vi "OpenStringFormatter Example.vi"() -> ()   [LabVIEW 2020]
uses:
  _built_ppls/OpenStringFormatter.lvlibp/StringFormatter.lvclass
panel:
  out "Value 2":string
  out "Value":string
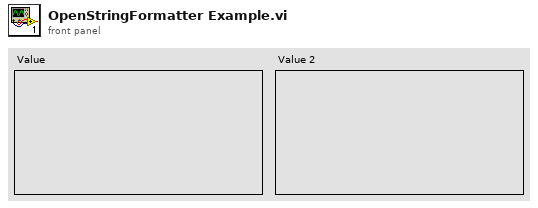
[diagram p1: front panel]
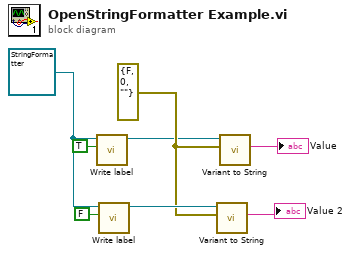
[diagram p0: block diagram]
diagram:
  w6 = errorcluster {"status"=FALSE, "code"=0, "source"=""} ("error constant")
  w4 = refnum<class "StringFormatter.lvclass"> refnum ("OpenStringFormatter.lvlibp:StringFormatter.lvclass")
  n1 = call "Write label.vi"("label"=TRUE, "StringFormatter in"=w4) -> ("StringFormatter out"=w3:refnum<class "StringFormatter.lvclass">)  [unwired: 9 in]
  n2 = call "Write label.vi"("label"=FALSE, "StringFormatter in"=w4) -> ("StringFormatter out"=w7:refnum<class "StringFormatter.lvclass">)  [unwired: 9 in]
  n3 = call "Variant to String.vi"("Variant"=w6, "StringFormatter in"=w7) -> ("Value"=→"Value 2":string)  [unwired: 7 in, 2 out]
  n4 = call "Variant to String.vi"("Variant"=w6, "StringFormatter in"=w3) -> ("Value"=→"Value":string)  [unwired: 7 in, 2 out]
